vi "Trafik Işığı.vi"() -> ()   [LabVIEW 2014]
panel:
  in  "stop":bool
  out "Y":bool
  out "S":bool
  out "K":bool
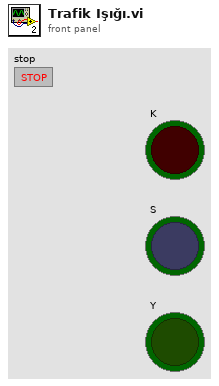
[diagram p1: front panel]
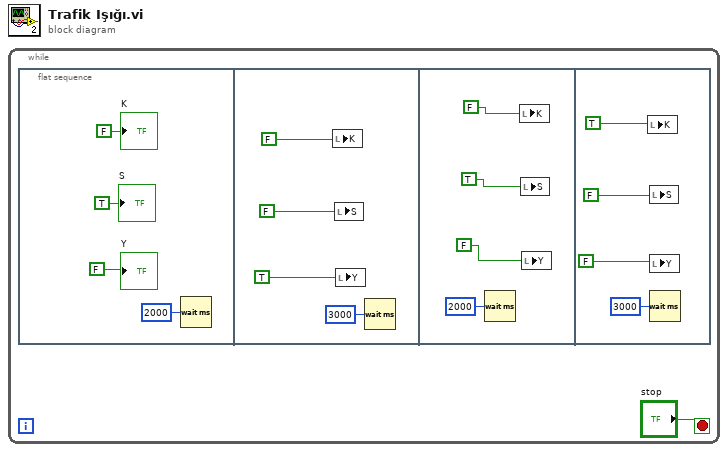
[diagram p0: block diagram]
diagram:
  n1 = while {
    stop <- "stop" stop-if-true
    n2 = flat-sequence {
      frame #0 {
        n3 = Wait (ms)(milliseconds to wait=u32 2000) -> ()  [unwired: 1 out]
        "K" <- FALSE
        "S" <- TRUE
        "Y" <- FALSE
      }
      frame #1 {
        n4 = local write "K"(FALSE) -> ()
        n5 = local write "S"(FALSE) -> ()
        n6 = local write "Y"(TRUE) -> ()
        n7 = Wait (ms)(milliseconds to wait=u32 3000) -> ()  [unwired: 1 out]
      }
      frame #2 {
        n8 = Wait (ms)(milliseconds to wait=u32 2000) -> ()  [unwired: 1 out]
        n9 = local write "K"(FALSE) -> ()
        n10 = local write "S"(TRUE) -> ()
        n11 = local write "Y"(FALSE) -> ()
      }
      frame #3 {
        n12 = local write "K"(TRUE) -> ()
        n13 = local write "S"(FALSE) -> ()
        n14 = local write "Y"(FALSE) -> ()
        n15 = Wait (ms)(milliseconds to wait=u32 3000) -> ()  [unwired: 1 out]
      }
    }
  }
